vi "accumulator.vi"(6 "first time":bool=TRUE, 7 "size":i32=1, 11 "number":dbl) -> (2 "mean":dbl)   [LabVIEW 2010]
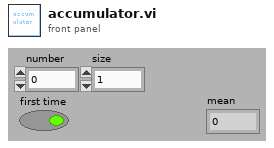
[diagram p1: front panel]
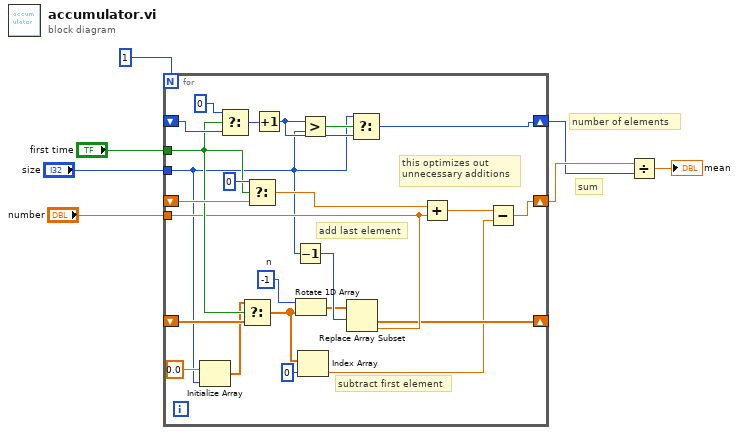
[diagram p0: block diagram]
diagram:
  # "sum"
  # "number of elements"
  n1 = for {
    N: 1 -> [_]
    tunnel: "first time" -> [w22]
    shift-right: [w14] -> w3
    shift-left: _ -> [w26]
    shift-right: [w28] -> w2
    shift-left: _ -> [w30]
    tunnel: "size" -> [w8]
    tunnel: "number" -> [w19]
    shift-right: [w16] -> _
    shift-left: _ -> [w21]
    w20 = -1  # n
    # "add last element"
    # "subtract first element"
    # "this optimizes out \nunnecessary additions"
    n2 = Initialize Array(0.0, w8) -> (w9:dbl[])
    n3 = Select(t=0, s=w22, f=w30) -> (s? t:f=w24:i32)
    n4 = Select(t=w9, s=w22, f=w21) -> (s? t:f=w12:dbl[])
    n5 = Select(t=0, s=w22, f=w26) -> (s? t:f=w25:dbl)
    n6 = Increment(x=w24) -> (x+1=w23:i32)
    n7 = Decrement(x=w8) -> (x-1=w18:i32)
    n8 = Rotate 1D Array(1:w12, 2:w20) -> (0:w17:dbl[])
    n9 = Index Array(array=w12, index=0) -> (element=w11:dbl)
    n10 = Greater?(x=w23, y=w8) -> (0:w29:bool)
    n11 = Replace Array Subset(array=w17, new element=w19, index=w18) -> (w16:dbl[])
    n12 = Select(t=w8, s=w29, f=w23) -> (s? t:f=w28:i32)
    n13 = Add(x=w25, y=w19) -> (x+y=w15:dbl)
    n14 = Subtract(x=w15, y=w11) -> (x-y=w14:dbl)
  }
  n15 = Divide(x=w3, y=w2) -> (x/y=→"mean":dbl)
